vi "Day 10.1 - discard corrupted.vi"(11 "input":string[](array[string])) -> (3 "output":i32)   [LabVIEW 2021]
panel:
  out "Mismatched close":string[](array[string])
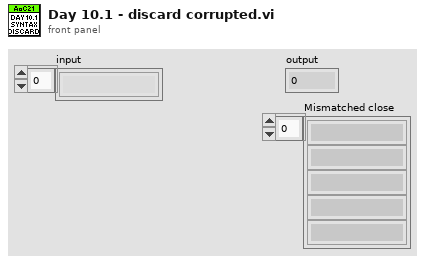
[diagram p1: front panel]
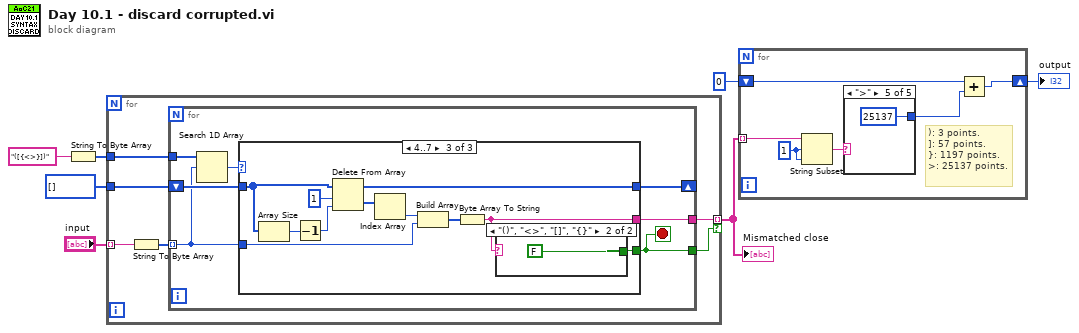
[diagram p0: block diagram]
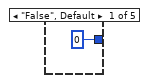
[diagram p2: hidden frame]
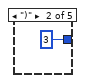
[diagram p3: hidden frame]
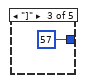
[diagram p4: hidden frame]
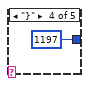
[diagram p5: hidden frame]
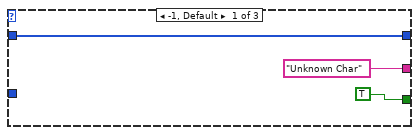
[diagram p6: hidden frame]
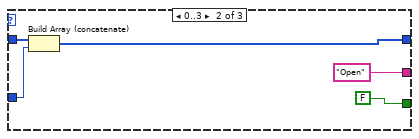
[diagram p7: hidden frame]
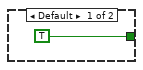
[diagram p8: hidden frame]
diagram:
  n1 = String To Byte Array(string="([{<>}])" ("regular expression")) -> (unsigned byte array=w4:u8[])
  n2 = for {
    tunnel: "input" -> [w11] mode=indexing
    tunnel: i32[] [] -> [w13]
    tunnel: w4 -> [w12]
    tunnel: [w9] -> w3 mode=indexing if=w8
    n3 = String To Byte Array(string=w11) -> (unsigned byte array=w10:u8[])
    n4 = for {
      shift-right: [w17] -> _
      shift-left: w13 -> [w18]
      tunnel: w12 -> [w20]
      tunnel: w10 -> [w16] mode=indexing
      tunnel: [w15] -> w9
      tunnel: [w14] -> w8
      stop <- w14 stop-if-true
      n5 = Search 1D Array(1D array=w20, element=w16) -> (index of element=w19:i32)  [unwired: 1 in]
      n6 = case shown="4..7" w19 {
        tunnel: [w23 w26 w35] -> w17
        tunnel: w18 -> [w23 w28 w36]
        tunnel: w16 -> [_ w27 w32]
        tunnel: [TRUE FALSE w29] -> w14
        tunnel: ["Unknown Char" ("string") "Open" ("string") w30] -> w15
        frame -1, Default {
        }
        frame 0..3 {
          n7 = Build Array (concatenate)(w28, w27) -> (w26:i32[])
        }
        frame 4..7 {
          n8 = Array Size(array=w36) -> (size(s)=w39:i32)
          n9 = Decrement(x=w39) -> (x-1=w38:i32)
          n10 = Delete From Array(array=w36, length=1, index=w38) -> (deleted portion=w34:i32[], array with subset deleted=w35:i32[])
          n11 = Index Array(array=w34) -> (element=w33:i32)  [unwired: 1 in]
          n12 = Build Array(w33, w32) -> (w31:i32[])
          n13 = Byte Array To String(unsigned byte array=w31) -> (string=w30:string)
          n14 = case shown="\"()\", \"<>\", \"[]\", \"{}\"" w30 {
            tunnel: [TRUE FALSE] -> w29
            frame Default {
            }
            frame "()", "<>", "[]", "{}" {
            }
          }
        }
      }
    }
  }
  "Mismatched close" <- w3
  n15 = for {
    tunnel: w3 -> [w47] mode=indexing
    shift-right: [w42] -> w1
    shift-left: 0 -> [w44]
    w46 = 1 ("offset (0)")
    # "): 3 points.\n]: 57 points.\n}: 1197 points.\n>: 25137 points."
    n16 = String Subset(string=w47, offset (0)=w46, length (rest)=w46) -> (substring=w45:string)
    n17 = case shown="\">\"" w45 {
      tunnel: [0 3 57 1197 25137] -> w43
      frame "False", Default {
      }
      frame ")" {
      }
      frame "]" {
      }
      frame "}" {
      }
      frame ">" {
      }
    }
    n18 = Add(x=w44, y=w43) -> (x+y=w42:i32)
  }
  "output" <- w1
